vi "Diag_GetEntityLocation.vi"(0 "GEA2 Reference In":refnum<k24>, 5 "GEA Inputs":T1={"Source"=228, "Destination"=0} {"Destination" format="%.0x"; "Source" format="%.0x"}, 7 "ERD Number from ERD 0x90":u16 format="%.0x", 11 "Error In":errorcluster) -> (4 "GEA2 Reference Out":refnum<k24>, 6 "Diagnostics Entity Location":u16 format="%.0x", 15 "Error Out":errorcluster)   [LabVIEW 2023]
uses:
  D:/Common/LabVIEW GEA2 Toolkit/source/GEA3 DLL Source/GeaCommunication.dll
  LabVIEW GEA2 Toolkit/source/GEA3 DLL Source/GeaCommunication.dll
  LabVIEW GEA2 Toolkit/GEA3/type defs/Source_Destination.ctl
  LabVIEW GEA2 Toolkit/GEA3/type defs/ERD Read Data In.ctl
  LabVIEW GEA2 Toolkit/GEA3/library/GEA2_Toolkit.lvlib
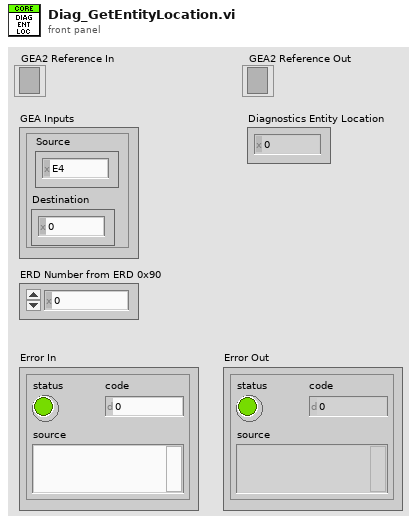
[diagram p1: front panel]
types:
  T1 = typedef "Source_Destination.ctl" = cluster{"Source":u8, "Destination":u8}
  T2 = typedef "ERD Read Data In.ctl" = cluster{"ERD Number":u16, "Data Type":enum16{"string", "boolean", "uint8_t", "uint16_t", "uint32_t", "uint64_t", "int8_t", "int16_t", "int32_t", "int64_t"}}
  T3 = typedef "ERD Read Data Out.ctl" = cluster{"ERD Number":u16, "Data":string}
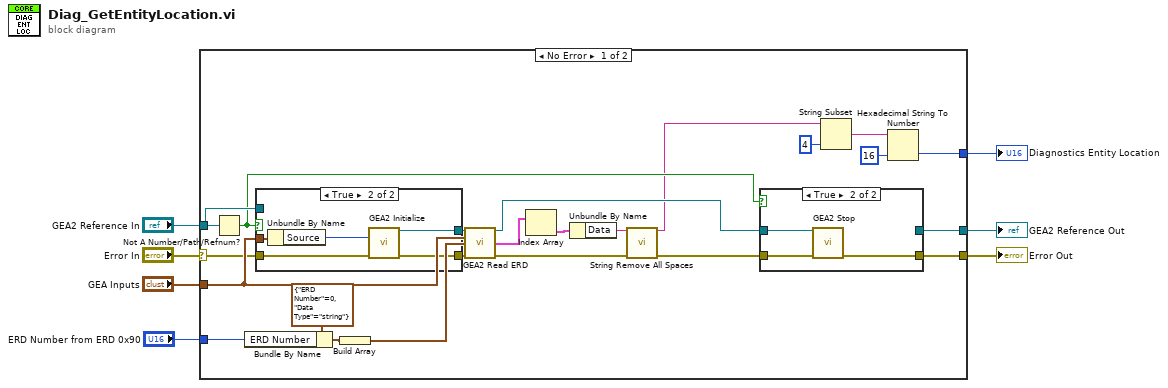
[diagram p0: block diagram]
diagram:
  n1 = case shown="No Error" "Error In" {
    selector: "Error In" -> [w18 w44]
    tunnel: [w17 w44] -> w7
    tunnel: "GEA2 Reference In" -> [w30 w43]
    tunnel: "GEA Inputs" -> [w23 _]
    tunnel: [w19 w43] -> w4
    tunnel: [w12 _] -> w2
    tunnel: "ERD Number from ERD 0x90" -> [w9 _]
    frame No Error {
      n2 = Not A Number/Path/Refnum?(number/path/refnum=w30) -> (NaN/Path/Refnum?=w20:bool)
      n3 = Bundle By Name(cluster=T2 {"ERD Number"=0, "Data Type"=enum."string"} ("ERD Read Data In"), "ERD Number"=w9) -> (w10:T2)
      n4 = case shown="True" w20 {
        tunnel: w18 -> [w36 w42]
        tunnel: w23 -> [_ w41]
        tunnel: [w36 w40] -> w28
        tunnel: [w37 w39] -> w27
        tunnel: w30 -> [w37 _]
        frame False {
        }
        frame True {
          n5 = Unbundle By Name(w41) -> ("Source"=w38:u8)
          n6 = call "GEA2 Initialize.vi"("Source Address"=w38, "error in"=w42) -> ("GEA2 Reference Out"=w39:refnum<k24>, "error out"=w40:errorcluster)  [unwired: 10 in, 2 out]
        }
      }
      n7 = Build Array(w10) -> (w8:T2[])
      n8 = call "GEA2 Read ERD.vi"("GEA2 Reference In"=w27, "GEA Inputs"=w23, "Read ERD List"=w8, "Error In"=w28) -> ("GEA2 Reference Out"=w21:refnum<k24>, "ERD Data Out"=w25:T3[], "Error Out"=w26:errorcluster)  [unwired: 8 in, 1 out]
      n9 = Index Array(array=w25) -> (element=w24:T3)  [unwired: 1 in]
      n10 = Unbundle By Name(w24) -> ("Data"=w29:string)
      n11 = call "String Remove All Spaces.vi"("Input String"=w29, "error in (no error)"=w26) -> ("Spaces Removed"=w13:string, "error out"=w22:errorcluster)  [unwired: 12 in]
      n12 = case shown="True" w20 {
        tunnel: w22 -> [w31 w35]
        tunnel: [w31 w34] -> w17
        tunnel: [w32 _] -> w19
        tunnel: w21 -> [w32 w33]
        frame False {
        }
        frame True {
          n13 = call "GEA2 Stop.vi"("GEA2 Reference In"=w33, "Error In"=w35) -> ("Error Out"=w34:errorcluster)  [unwired: 13 in]
        }
      }
      n14 = String Subset(string=w13, length (rest)=4 ("length (rest)")) -> (substring=w15:string)  [unwired: 1 in]
      n15 = Hexadecimal String To Number(string=w15, default (0uL)=u16 16 ("default (0 U32)")) -> (number=w12:u16)  [unwired: 1 in, 1 out]
    }
    frame Error {
    }
  }
  "Error Out" <- w7
  "GEA2 Reference Out" <- w4
  "Diagnostics Entity Location" <- w2
